vi "Tosca-Validate Sequence Expressions.vi"(0 "Family in":T1, 11 "error in (no error)":errorcluster) -> (4 "Family out":T1, 15 "error out":errorcluster)   [LabVIEW 2020]
uses:
  Typedefs/Tosca-Parameter Family.ctl
  Typedefs/Tosca-Parameter Table Element.ctl
  Typedefs/Tosca-Parameter Dimension.ctl
  Typedefs/Tosca-Family Order.ctl
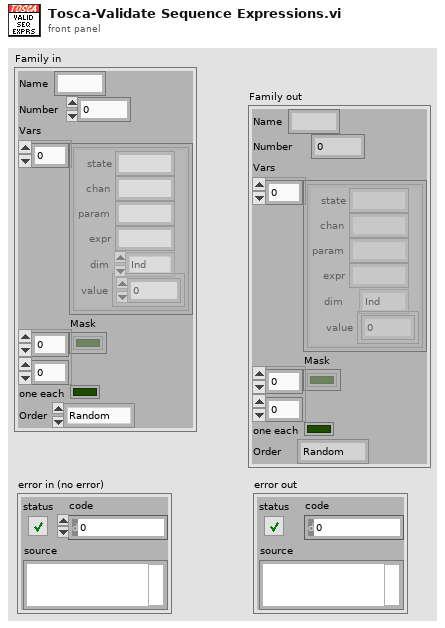
[diagram p1: front panel]
types:
  T1 = typedef "Tosca-Parameter Family.ctl" = cluster{"Name":string, "Number":i32, "Vars":T2[], "Mask":bool[][], "one each":bool, "Order":T4}
  T2 = typedef "Tosca-Parameter Table Element.ctl" = cluster{"state":string, "chan":string, "param":string, "expr":string, "dim":T3, "value":dbl[]}
  T3 = typedef "Tosca-Parameter Dimension.ctl" = enum16{"Ind", "X", "Y"}
  T4 = typedef "Tosca-Family Order.ctl" = enum16{"Random", "Sequential"}
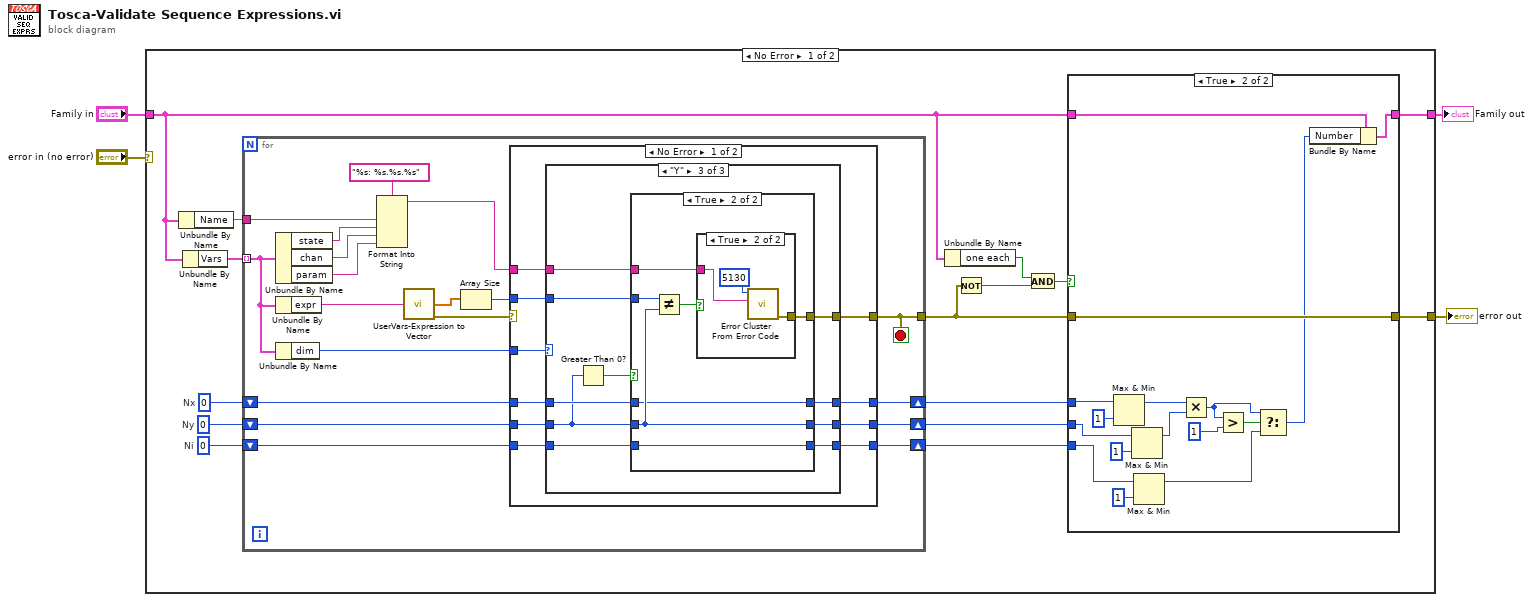
[diagram p0: block diagram]
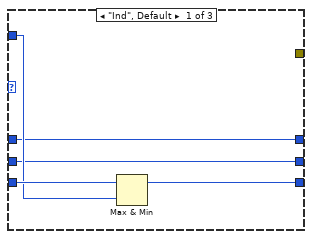
[diagram p3: hidden frame]
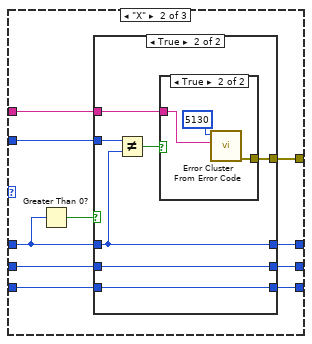
[diagram p4: hidden frame]
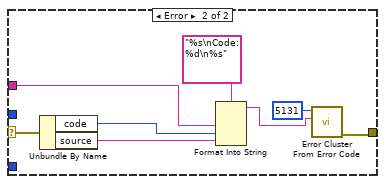
[diagram p9: hidden frame]
diagram:
  n1 = case shown="No Error" "error in (no error)" {
    selector: "error in (no error)" -> [_ w126]
    tunnel: "Family in" -> [w10 w127]
    tunnel: [w13 w127] -> w3
    tunnel: [w14 w126] -> w1
    frame No Error {
      w15 = 0  # Ni
      w16 = 0  # Ny
      w18 = 0  # Nx
      n2 = Unbundle By Name(w10) -> ("Name"=w17:string)
      n3 = Unbundle By Name(w10) -> ("Vars"=w19:T2[])
      n4 = for {
        tunnel: w19 -> [w47] mode=indexing
        shift-right: [w50] -> w7
        shift-left: w18 -> [w51]
        tunnel: w17 -> [w48]
        tunnel: [w42] -> w12
        shift-right: [w40] -> w6
        shift-left: w16 -> [w41]
        shift-right: [w38] -> w5
        shift-left: w15 -> [w39]
        stop <- w42 stop-if-true
        n5 = Unbundle By Name(w47) -> ("state"=w46:string, "chan"=w45:string, "param"=w44:string)
        n6 = Unbundle By Name(w47) -> ("expr"=w56:string)
        n7 = Unbundle By Name(w47) -> ("dim"=w52:T3)
        n8 = Format Into String(format string="%s: %s.%s.%s", w48, w46, w45, w44) -> (resulting string=w43:string)  [unwired: 2 in, 1 out]
        n9 = call "UserVars-Expression to Vector.vi"("Expr"=w56) -> ("Values"=w54:dbl[], "error out"=w55:errorcluster)  [unwired: 13 in]
        n10 = Array Size(array=w54) -> (size(s)=w53:i32)
        n11 = case shown="No Error" w55 {
          selector: w55 -> [_ w123]
          tunnel: w53 -> [w65 _]
          tunnel: w52 -> [w66 _]
          tunnel: w51 -> [w64 _]
          tunnel: [w63 _] -> w50
          tunnel: [w62 w125] -> w42
          tunnel: w43 -> [w61 w121]
          tunnel: w41 -> [w60 _]
          tunnel: [w59 _] -> w40
          tunnel: w39 -> [w58 _]
          tunnel: [w57 _] -> w38
          frame No Error {
            n12 = case shown="\"Y\"" w66 {
              tunnel: w65 -> [w70 w80 w103]
              tunnel: w64 -> [w68 w79 w102]
              tunnel: [w68 w78 w101] -> w63
              tunnel: [_ w77 w100] -> w62
              tunnel: w61 -> [_ w76 w99]
              tunnel: w60 -> [w67 w75 w95]
              tunnel: [w67 w74 w98] -> w59
              tunnel: w58 -> [w71 w72 w96]
              tunnel: [w69 w73 w97] -> w57
              frame "Ind", Default {
                n13 = Max & Min(x=w71, y=w70) -> (max(x,y)=w69:i32)  [unwired: 1 out]
              }
              frame "X" {
                n14 = Greater Than 0?(x=w79) -> (x > 0?=w81:bool)
                n15 = case shown="True" w81 {
                  tunnel: w80 -> [w84 w91]
                  tunnel: w79 -> [_ w86]
                  tunnel: [w84 w86] -> w78
                  tunnel: [_ w89] -> w77
                  tunnel: w76 -> [_ w88]
                  tunnel: w75 -> [w83 w87]
                  tunnel: [w83 w87] -> w74
                  tunnel: [w82 w85] -> w73
                  tunnel: w72 -> [w82 w85]
                  frame False {
                  }
                  frame True {
                    n16 = Not Equal?(x=w91, y=w86) -> (x != y?=w90:bool)
                    n17 = case shown="True" w90 {
                      tunnel: [_ w94] -> w89
                      tunnel: w88 -> [_ w93]
                      frame False {
                      }
                      frame True {
                        n18 = call <vilib>:"Error Cluster From Error Code.vi"("error message (\"\")"=w93, "error code (0)"=5130) -> ("error out"=w94:errorcluster)  [unwired: 7 in]
                      }
                    }
                  }
                }
              }
              frame "Y" {
                n19 = Greater Than 0?(x=w95) -> (x > 0?=w104:bool)
                n20 = case shown="True" w104 {
                  tunnel: w103 -> [w106 w114]
                  tunnel: w102 -> [w107 w109]
                  tunnel: [w107 w109] -> w101
                  tunnel: [_ w112] -> w100
                  tunnel: w99 -> [_ w111]
                  tunnel: w95 -> [_ w110]
                  tunnel: [w106 w110] -> w98
                  tunnel: [w105 w108] -> w97
                  tunnel: w96 -> [w105 w108]
                  frame False {
                  }
                  frame True {
                    n21 = Not Equal?(x=w114, y=w110) -> (x != y?=w113:bool)
                    n22 = case shown="True" w113 {
                      tunnel: [_ w117] -> w112
                      tunnel: w111 -> [_ w116]
                      frame False {
                      }
                      frame True {
                        n23 = call <vilib>:"Error Cluster From Error Code.vi"("error message (\"\")"=w116, "error code (0)"=5130) -> ("error out"=w117:errorcluster)  [unwired: 7 in]
                      }
                    }
                  }
                }
              }
            }
          }
          frame Error {
            n24 = Unbundle By Name(w123) -> ("code"=w120:i32, "source"=w119:string)
            n25 = Format Into String(format string="%s\nCode: %d\n%s", w121, w120, w119) -> (resulting string=w118:string)  [unwired: 2 in, 1 out]
            n26 = call <vilib>:"Error Cluster From Error Code.vi"("error message (\"\")"=w118, "error code (0)"=5131) -> ("error out"=w125:errorcluster)  [unwired: 7 in]
          }
        }
      }
      n27 = Unbundle By Name(w10) -> ("one each"=w9:bool)
      n28 = Not(x=w12) -> (.not. x?=w11:bool)
      n29 = And(x=w9, y=w11) -> (x .and. y?=w8:bool)
      n30 = case shown="True" w8 {
        tunnel: [w20 w37] -> w14
        tunnel: w10 -> [w21 w36]
        tunnel: [w21 w35] -> w13
        tunnel: w12 -> [w20 w37]
        tunnel: w7 -> [_ w34]
        tunnel: w6 -> [_ w31]
        tunnel: w5 -> [_ w23]
        frame False {
        }
        frame True {
          n31 = Max & Min(x=w34, y=1) -> (max(x,y)=w30:i32)  [unwired: 1 out]
          n32 = Max & Min(x=w31, y=1) -> (max(x,y)=w29:i32)  [unwired: 1 out]
          n33 = Max & Min(x=w23, y=1) -> (max(x,y)=w22:i32)  [unwired: 1 out]
          n34 = Multiply(x=w30, y=w29) -> (x*y=w26:i32)
          n35 = Greater?(x=w26, y=1) -> (0:w27:bool)
          n36 = Select(t=w26, s=w27, f=w22) -> (s? t:f=w25:i32)
          n37 = Bundle By Name(cluster=w36, "Number"=w25) -> (w35:T1)
        }
      }
    }
    frame Error {
    }
  }
  "error out" <- w1
  "Family out" <- w3
